vi "Read Config Files Directory.vi"(8 "error in (no error)":errorcluster, 11 "Config Manager Class in":refnum<class "Config Manager.lvclass">) -> (0 "error out":errorcluster, 2 "Config Files Directory":path, 3 "Config Manager Class out":refnum<class "Config Manager.lvclass">)   [LabVIEW 2017, in "Config Manager.lvclass"]
uses:
  Config Manager.lvclass
  Config Manager.lvclass/Config Manager.ctl
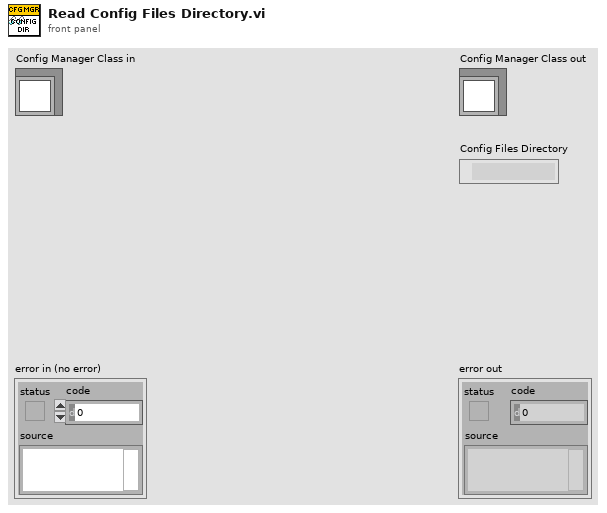
[diagram p1: front panel]
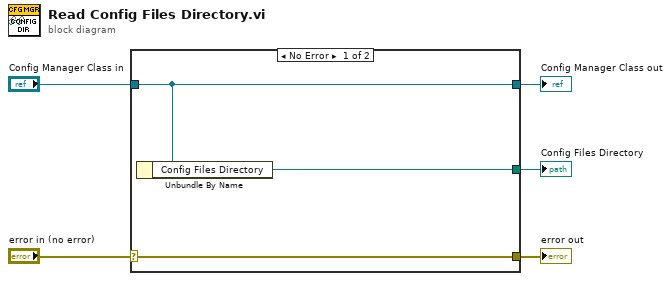
[diagram p0: block diagram]
diagram:
  n1 = case shown="No Error" "error in (no error)" {
    selector: "error in (no error)" -> [w8 w9]
    tunnel: [w8 w9] -> w4
    tunnel: [w7 w10] -> w2
    tunnel: "Config Manager Class in" -> [w7 w10]
    tunnel: [w6 _] -> w1
    frame No Error {
      n2 = Unbundle By Name(w7) -> ("Config Files Directory"=w6:path)
    }
    frame Error {
    }
  }
  "error out" <- w4
  "Config Manager Class out" <- w2
  "Config Files Directory" <- w1
